vi "Image.vi"(2 "XRef":refnum<vi>, 3 "State In":T1={"Enum Type"=variant(dbl 0.0), "Types Type"=variant, "Enum Names"=[], "Type Names"=[], "Typedef Name"="", "Typedef Path"=path ""}) -> (0 "Image":picture)   [LabVIEW 2015, in "Define-Tagged-Union.xnode"]
doc: "This ability VI is used to describe your XNode's appearance. The origin of Image corresponds to the top-left corner of your XNode. The bounds of your XNode are used to crop this image. If you want LabVIEW to update your image, you need to inform it through the UpdateImage or UpdateImageAndBounds replies. Any areas where you do not draw are transparent, so regions intended to appear white should be explicitly drawn.\n \n Remember to localize any strings that are part of your image.\n\nDefault behavior: None.\n\nThis ability does not provide UI and OS messages are not handled."
uses:
  Define-Tagged-Union.xnode
  State.ctl
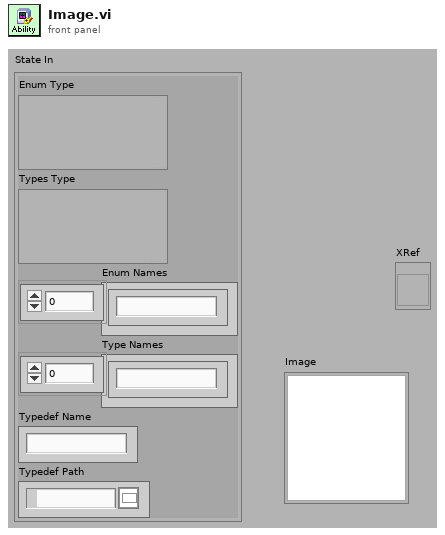
[diagram p1: front panel]
types:
  T1 = typedef "Define-Tagged-Union.xnode/State.ctl" = cluster{"Enum Type":variant, "Types Type":variant, "Enum Names":string[], "Type Names":string[], "Typedef Name":string, "Typedef Path":path}
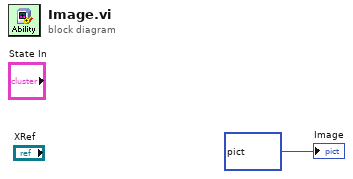
[diagram p0: block diagram]
diagram:
  "Image" <- picture bytes[4638] ("Image 2")
